vi "message.vi"(1 "itemlist":string[][](array[string]), 2 "item":string[](array[string])) -> (0 "itemlistout":string[][](array[string]))   [LabVIEW 2015]
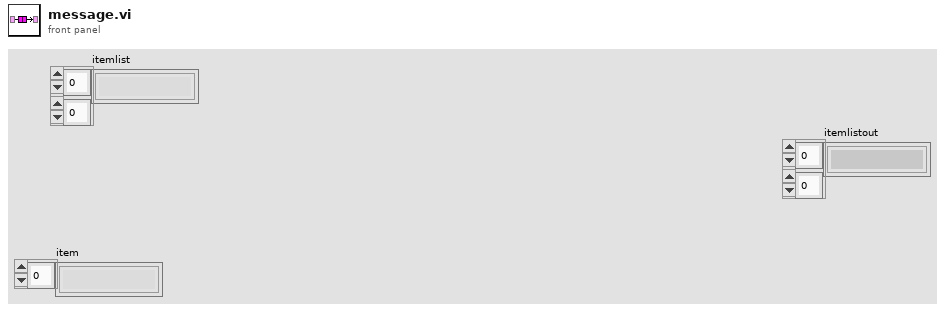
[diagram p1: front panel]
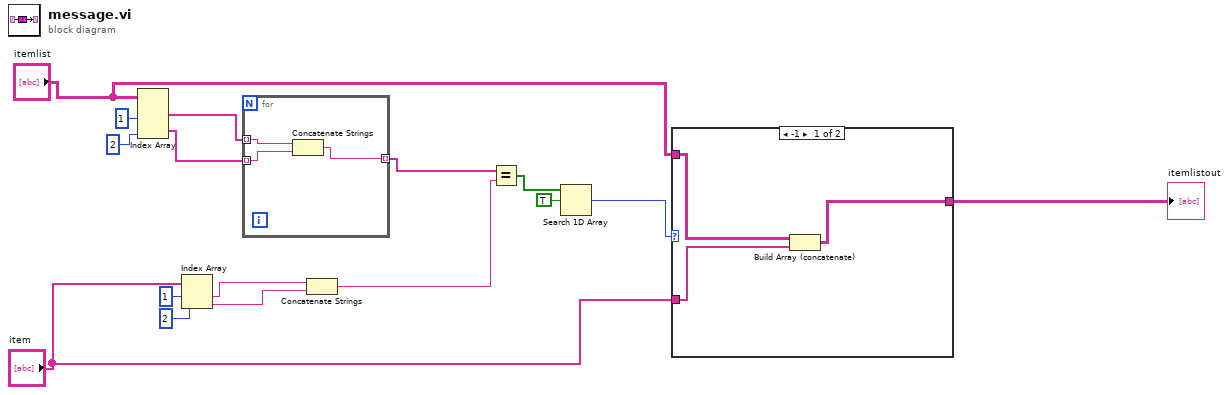
[diagram p0: block diagram]
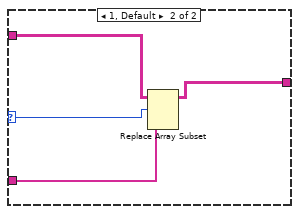
[diagram p2: hidden frame]
diagram:
  n1 = Index Array(array="itemlist", index (col) #1=1 ("禁用的索引 (列)"), index (col) #2=2 ("索引 (列)")) -> (element #1=w14:string[], element #2=w13:string[])  [unwired: 2 in]
  n2 = Index Array(array="item", index #1=1 ("索引"), index #2=2 ("索引")) -> (element #1=w9:string, element #2=w8:string)
  n3 = for {
    tunnel: w14 -> [w19] mode=indexing
    tunnel: w13 -> [w18] mode=indexing
    tunnel: [w17] -> w12 mode=indexing
    n4 = Concatenate Strings(w19, w18) -> (w17:string)
  }
  n5 = Concatenate Strings(w9, w8) -> (w7:string)
  n6 = Equal?(x=w12, y=w7) -> (x = y?=w6:bool[])
  n7 = Search 1D Array(1D array=w6, element=TRUE ("元素")) -> (index of element=w4:i32)  [unwired: 1 in]
  n8 = case shown="-1" w4 {
    selector: w4 -> [_ w25]
    tunnel: "itemlist" -> [w22 w26]
    tunnel: "item" -> [w21 w24]
    tunnel: [w20 w23] -> w1
    frame -1 {
      n9 = Build Array (concatenate)(w22, w21) -> (w20:string[][])
    }
    frame 1, Default {
      n10 = Replace Array Subset(array=w26, new element=w24, index (row)=w25) -> (w23:string[][])  [unwired: 1 in]
    }
  }
  "itemlistout" <- w1
